vi "Get Cluster Items and Values.vi"(8 "Error In":errorcluster, 11 "Generic Cluster Reference":refnum<vi>) -> (0 "Error Out":errorcluster, 1 "String Values":string[](array[string]), 2 "Column":string[](array[string]), 3 "Database":string)   [LabVIEW 2018, in "Database.lvlib"]
uses:
  Database.lvlib
  <vilib>/Utility/Data Type/Type Definitions/Data Type.ctl
  <vilib>/Utility/Data Type/NI_Data Type.lvlib
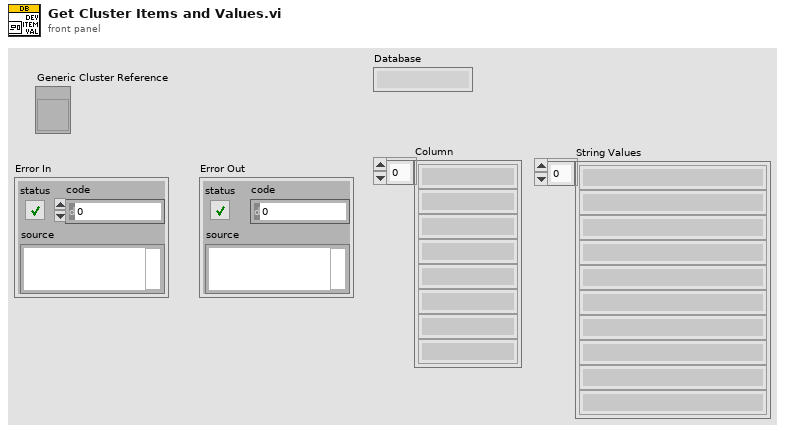
[diagram p1: front panel]
types:
  T1 = typedef "NI_Data Type.lvlib/Data Type.ctl" = enum8{"Invalid Type", "Void", "I8", "I16", "I32", "I64", "U8", "U16", "U32", "U64", "Single Float", "Double Float", "Extended Float", "Single Complex", "Double Complex", "Extended Complex", "Enum U8", "Enum U16", "Enum U32", "Enum U64", "Single Float With Unit", "Double Float With Unit", "Extended Float With Unit", "Single Complex with Unit", "Double Complex with Unit", "Extended Complex with Unit", "Boolean", "String", "Path", "Picture", "Tag", "Array", "Cluster", "Variant", "LV Variant", "Waveform", "Timestamp", "Digital Waveform", "Digital Data", "ExpressData", "Refnum", "External Data", "VI", "Poly VI", "LabVIEW Class Instance", "Fixed Point"}
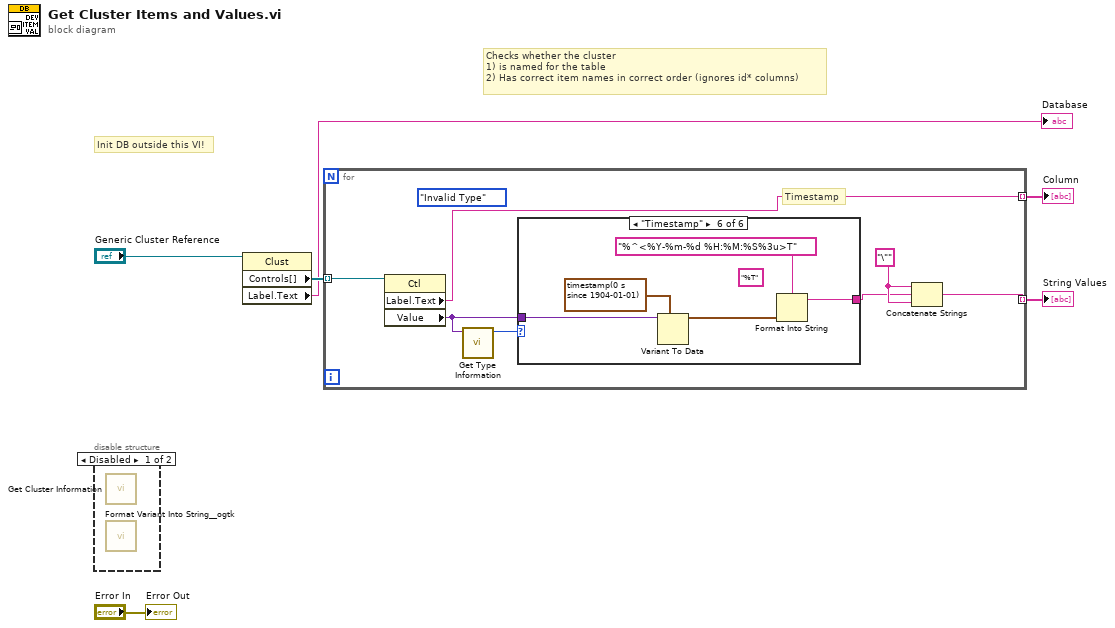
[diagram p0: block diagram]
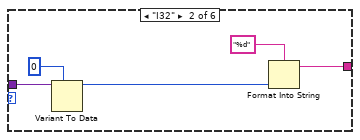
[diagram p4: hidden frame]
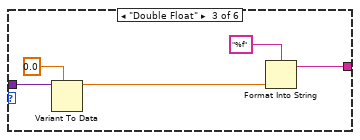
[diagram p5: hidden frame]
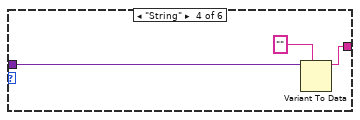
[diagram p6: hidden frame]
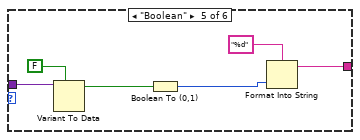
[diagram p7: hidden frame]
diagram:
  # "Init DB outside this VI!"
  # "Checks whether the cluster \n1) is named for the table\n2) Has correct item names in correct order (ignores id* columns)"
  n1 = disable-structure shown="Disabled" {
    frame Disabled {
      n2 = call <vilib>:"Get Cluster Information.vi"() -> ()  [unwired: 10 in, 2 out]
      n3 = call <userlib>:"Format Variant Into String__ogtk.vi"() -> ()  [unwired: 14 in, 2 out]
    }
    frame Enabled {
    }
  }
  n4 = property class="Clust"(reference="Generic Cluster Reference") -> ("Controls[]"=w5:refnum<vi>[], "Label.Text"=→"Database":string)  [unwired: 1 in, 2 out]
  n5 = for {
    tunnel: w5 -> [w13] mode=indexing
    tunnel: [w12] -> w1 mode=indexing
    tunnel: [w7] -> w2 mode=indexing
    w9 = "\"" ("string")
    (unwired) Data_Type."Invalid Type" ("Type")
    # "Timestamp"
    n6 = property class="Ctl"(reference=w13) -> ("Label.Text"=w12:string, "Value"=w10:variant)  [unwired: 1 in, 2 out]
    n7 = call <vilib>:"Get Type Information.vi"("Variant"=w10) -> ("Type"=w11:T1)  [unwired: 6 in, 4 out]
    n8 = case shown="\"Timestamp\"" w11 {
      tunnel: w10 -> [_ w17 w22 w25 w31 w36]
      tunnel: [_ w14 w19 w24 w29 w34] -> w8
      frame Default {
      }
      frame "I32" {
        n9 = Variant To Data(type=0, Variant=w17) -> (data=w16:i32)  [unwired: 1 in, 1 out]
        n10 = Format Into String(format string="%d", w16) -> (resulting string=w14:string)  [unwired: 2 in, 1 out]
      }
      frame "Double Float" {
        n11 = Variant To Data(type=0.0, Variant=w22) -> (data=w21:dbl)  [unwired: 1 in, 1 out]
        n12 = Format Into String(format string="%f", w21) -> (resulting string=w19:string)  [unwired: 2 in, 1 out]
      }
      frame "String" {
        n13 = Variant To Data(type="", Variant=w25) -> (data=w24:string)  [unwired: 1 in, 1 out]
      }
      frame "Boolean" {
        n14 = Variant To Data(type=FALSE, Variant=w31) -> (data=w27:bool)  [unwired: 1 in, 1 out]
        n15 = Boolean To (0,1)(Boolean=w27) -> (0, 1=w28:i16)
        n16 = Format Into String(format string="%d", w28) -> (resulting string=w29:string)  [unwired: 2 in, 1 out]
      }
      frame "Timestamp" {
        (unwired) "%T" ("format string")
        n17 = Variant To Data(type=timestamp(0 s since 1904-01-01), Variant=w36) -> (data=w35:timestamp)  [unwired: 1 in, 1 out]
        n18 = Format Into String(format string="%^<%Y-%m-%d %H:%M:%S%3u>T", w35) -> (resulting string=w34:string)  [unwired: 2 in, 1 out]
      }
    }
    n19 = Concatenate Strings(w9, w8, w9) -> (w7:string)
  }
  "String Values" <- w2
  "Column" <- w1
  "Error Out" <- "Error In"
